vi "USBTC08Close.vi"(8 "error in (no error)":errorcluster, 11 "Handle in":i16) -> (0 "error out":errorcluster, 3 "handle":i16)   [LabVIEW 2010]
uses:
  usbtc08.dll
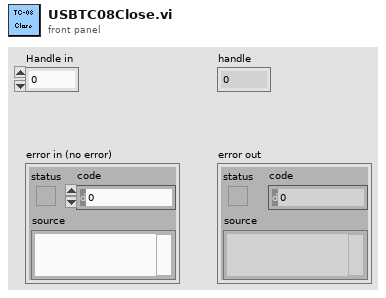
[diagram p1: front panel]
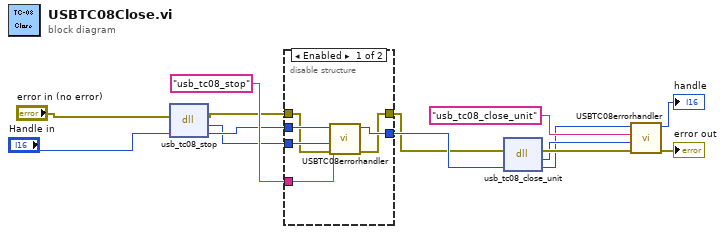
[diagram p0: block diagram]
diagram:
  n1 = dll-call lib="usbtc08.dll" fn="usb_tc08_stop" ("Close unit")(error in="error in (no error)", "handle"="Handle in") -> (error out=w7:errorcluster, "return type"=w10:i16, "handle"=w11:i16)  [unwired: 2 in, 1 out]
  n2 = disable-structure shown="Enabled" {
    disable-tunnel: "usb_tc08_stop" ("API function") -> [w20 _]
    disable-tunnel: w11 -> [w19 w22]
    disable-tunnel: [w18 w22] -> w9
    disable-tunnel: w10 -> [w17 _]
    disable-tunnel: [w16 w21] -> w8
    disable-tunnel: w7 -> [w15 w21]
    frame Enabled {
      n3 = call "USBTC08errorhandler.vi"("error in (no error)"=w15, "Return"=w17, "API function"=w20, "Handle in"=w19) -> ("error out"=w16:errorcluster, "Handle out"=w18:i16)  [unwired: 6 in]
    }
    frame Disabled {
    }
  }
  n4 = dll-call lib="usbtc08.dll" fn="usb_tc08_close_unit" ("Close unit")(error in=w8, "handle"=w9) -> (error out=w6:errorcluster, "return type"=w4:i16, "handle"=w3:i16)  [unwired: 2 in, 1 out]
  n5 = call "USBTC08errorhandler.vi"("error in (no error)"=w6, "Return"=w4, "API function"="usb_tc08_close_unit", "Handle in"=w3) -> ("error out"=→"error out":errorcluster, "Handle out"=→"handle":i16)  [unwired: 6 in]
